vi "Copy PPL for Target Type.vi"(6 "Top Level/Always Included VIs":path[](array[path]), 7 "Main Destination Path":path, 9 "Target Name":string, 10 "Build Specification Name":string, 11 "Project Path":path) -> (0 "error out":errorcluster)   [LabVIEW 2020]
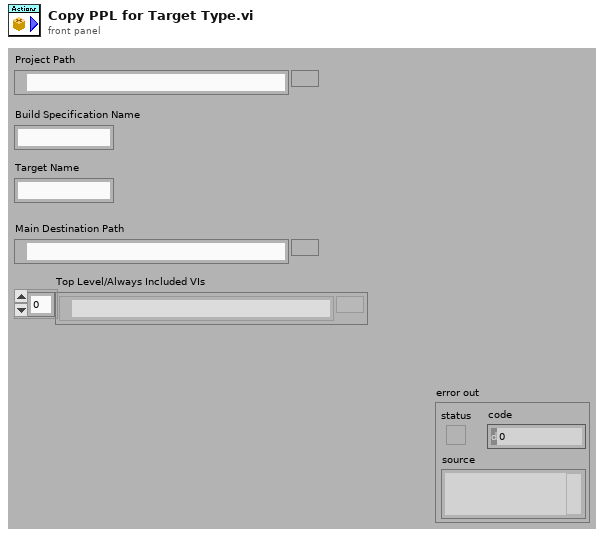
[diagram p1: front panel]
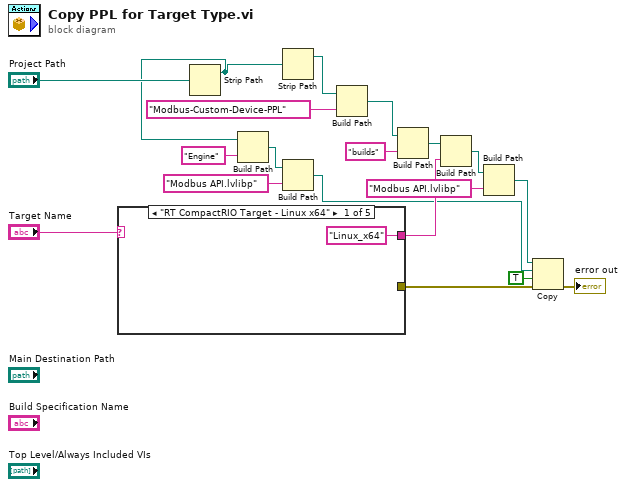
[diagram p0: block diagram]
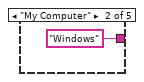
[diagram p2: hidden frame]
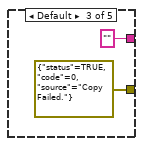
[diagram p3: hidden frame]
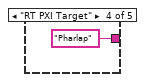
[diagram p4: hidden frame]
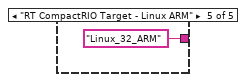
[diagram p5: hidden frame]
diagram:
  n1 = case shown="\"RT CompactRIO Target - Linux x64\"" "Target Name" {
    tunnel: ["Linux_x64" "Windows" "" "Pharlap" "Linux_32_ARM"] -> w17
    tunnel: [_ _ errorcluster {"status"=TRUE, "code"=0, "source"="Copy Failed."} ("error in") _ _] -> w2
    frame "RT CompactRIO Target - Linux x64" {
    }
    frame "My Computer" {
    }
    frame Default {
    }
    frame "RT PXI Target" {
    }
    frame "RT CompactRIO Target - Linux ARM" {
    }
  }
  n2 = Strip Path(path="Project Path") -> (stripped path=w12:path)  [unwired: 1 out]
  n3 = Build Path(base path=w12, name or relative path="Engine") -> (appended path=w9:path)
  n4 = Strip Path(path=w12) -> (stripped path=w16:path)  [unwired: 1 out]
  n5 = Build Path(base path=w9, name or relative path="Modbus API.lvlibp") -> (appended path=w4:path)
  n6 = Build Path(base path=w16, name or relative path="Modbus-Custom-Device-PPL") -> (appended path=w14:path)
  n7 = Build Path(base path=w14, name or relative path="builds") -> (appended path=w8:path)
  n8 = Build Path(base path=w8, name or relative path=w17) -> (appended path=w6:path)
  n9 = Build Path(base path=w6, name or relative path="Modbus API.lvlibp") -> (appended path=w5:path)
  n10 = Copy(8:w2, 9:TRUE ("overwrite (F)"), 10:w4, 11:w5) -> (0:→"error out":errorcluster)  [unwired: 1 in, 2 out]
